vi "Listen and reply broadcast.ping.vi"(2 "error (in)":errorcluster, 3 "driplineinfolocation":string, 4 "host name":string="higgsino.physics.ucsb.edu", 5 "service name":string="monitor") -> (0 "error out":errorcluster, 1 "Log":string)   [LabVIEW 2016]
uses:
  C:/Program Files (x86)/National Instruments/LabVIEW 2016/vi.lib/Distrio/LabbitMQ/RabbitMQ.Client.dll
  Program Files (x86)/National Instruments/LabVIEW 2016/vi.lib/Distrio/LabbitMQ/RabbitMQ.Client.dll
  <vilib>/Distrio/LabbitMQ/Queue/Queue.lvclass
  <vilib>/Distrio/LabbitMQ/Connection/Connection.lvclass
panel:
  in  "stop":bool
  in  "Tab Control":enum32{"AMQP Settings", "Logger"}(tab)
  out "binding keys":string[](array[string])
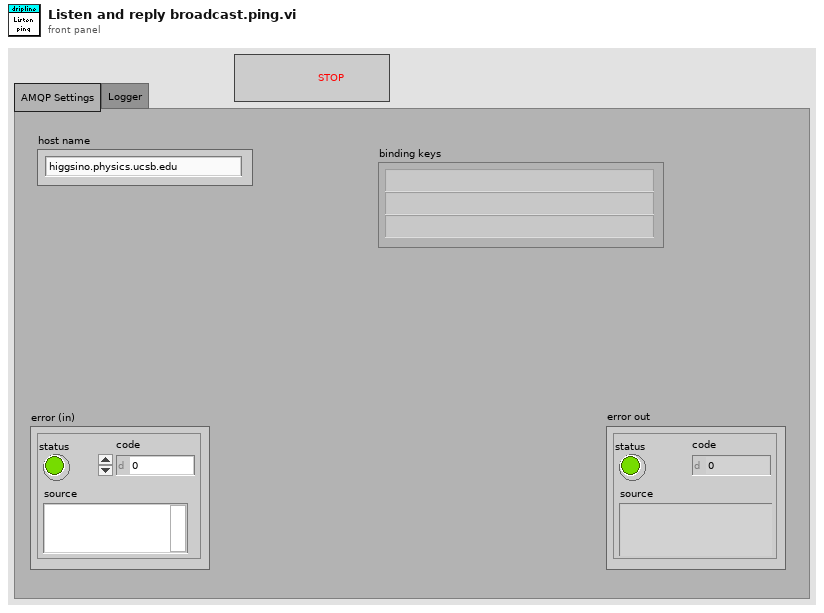
[diagram p1: front panel]
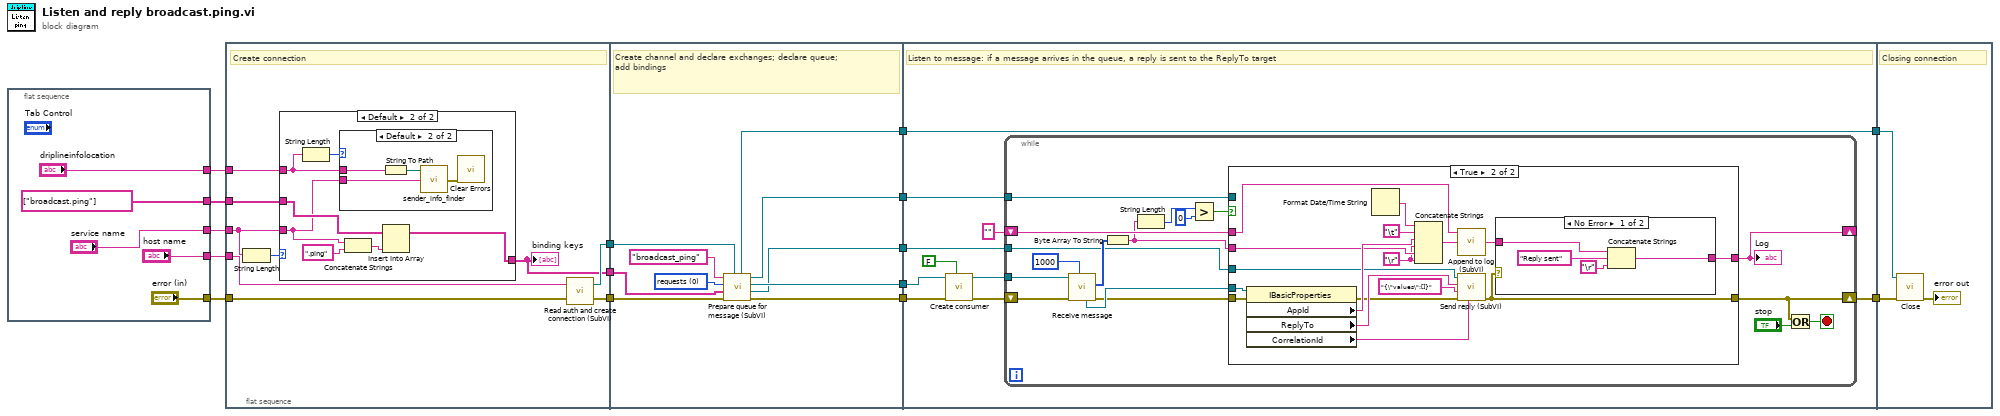
[diagram p0: block diagram]
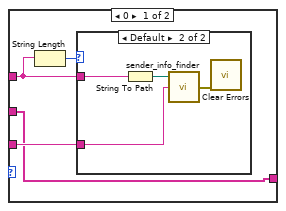
[diagram p2: hidden frame]
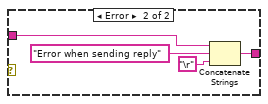
[diagram p6: hidden frame]
diagram:
  n1 = flat-sequence {
    tunnel: ["error (in)"] -> w13
    tunnel: ["host name"] -> w12
    tunnel: ["service name"] -> w4
    tunnel: ["driplineinfolocation"] -> w3
    tunnel: [string[] ["broadcast.ping"] ("broadcast.ping")] -> w1
    frame #0 {
    }
  }
  n2 = flat-sequence {
    tunnel: [w27] -> w15
    tunnel: [w26] -> w14
    tunnel: w12 -> [w29]
    tunnel: w13 -> [w28]
    tunnel: w4 -> [w24]
    tunnel: w3 -> [w25]
    tunnel: [w23] -> w2
    tunnel: w1 -> [w22]
    tunnel: w15 -> [w54]
    tunnel: w14 -> [w53]
    tunnel: [w56] -> w10
    tunnel: [w55] -> w9
    tunnel: [w52] -> w7
    tunnel: [w51] -> w6
    tunnel: [w50] -> w5
    tunnel: w2 -> [w49]
    tunnel: [w67] -> w11
    tunnel: w10 -> [w64]
    tunnel: w9 -> [w63]
    tunnel: [w62] -> w8
    tunnel: w7 -> [w62]
    tunnel: w6 -> [w61]
    tunnel: w5 -> [w60]
    tunnel: w11 -> [w114]
    tunnel: w8 -> [w113]
    frame #0 {
      # "Create connection"
      n3 = String Length(string=w24) -> (length=w21:i32)
      n4 = case shown="Default" w21 {
        tunnel: w25 -> [w30 w43]
        tunnel: w24 -> [w33 w38]
        tunnel: [w32 w40] -> w23
        tunnel: w22 -> [w32 w39]
        frame 0 {
          n5 = String Length(string=w30) -> (length=w31:i32)
          n6 = case shown="Default" w31 {
            tunnel: w33 -> [_ w37]
            tunnel: w30 -> [_ w34]
            frame 0 {
            }
            frame Default {
              n7 = String To Path(string=w34) -> (path=w36:path)
              n8 = call "sender_info_finder.vi"("service name"=w37, "file (use dialog)"=w36) -> ("error (out)"=w35:errorcluster)  [unwired: 1 in]
              n9 = call <vilib>:"Clear Errors.vi"("error in (no error)"=w35) -> ()  [unwired: 5 in, 2 out]
            }
          }
        }
        frame Default {
          n10 = String Length(string=w43) -> (length=w44:i32)
          n11 = case shown="Default" w44 {
            tunnel: w38 -> [_ w48]
            tunnel: w43 -> [_ w45]
            frame 0 {
            }
            frame Default {
              n12 = String To Path(string=w45) -> (path=w47:path)
              n13 = call "sender_info_finder.vi"("service name"=w48, "file (use dialog)"=w47) -> ("error (out)"=w46:errorcluster)  [unwired: 1 in]
              n14 = call <vilib>:"Clear Errors.vi"("error in (no error)"=w46) -> ()  [unwired: 5 in, 2 out]
            }
          }
          n15 = Concatenate Strings(w38, ".ping" ("string")) -> (w41:string)
          n16 = Insert Into Array(array=w39, new element=w41) -> (w40:string[])  [unwired: 1 in]
        }
      }
      "binding keys" <- w23
      n17 = call "Read auth and create connection (SubVI).vi"("error in (no error)"=w28, "host name"=w29) -> ("error out"=w26:errorcluster, "Connection out"=w27:refnum<class "Connection.lvclass">)
    }
    frame #1 {
      w57 = u16 0 items=["requests", "alerts"] ("exchange name")
      # "Create channel and declare exchanges; declare queue;\nadd bindings"
      n18 = call "Prepare queue for message (SubVI).vi"("Connection in"=w54, "error in (no error)"=w53, "binding key"=w49, "exchange name"=w57, "queue \nname"="broadcast_ping" ("queue name")) -> ("error out"=w55:errorcluster, "Exchange.lvclass"=w51:refnum<class "Exchange.lvclass">, "Queue out"=w56:refnum<class "Queue.lvclass">, "Channel out"=w50:refnum<class "Channel.lvclass">, "Connection out"=w52:refnum<class "Connection.lvclass">)
    }
    frame #2 {
      # "Listen to message: if a message arrives in the queue, a reply is sent to the ReplyTo target"
      n19 = call <vilib>:"Create consumer.vi"("noAck? (T)"=FALSE, "error in (no error)"=w63, "Queue in"=w64) -> ("error out"=w66:errorcluster, "Queue out"=w68:refnum<class "Queue.lvclass">)  [unwired: 7 in]
      n20 = while {
        tunnel: w68 -> [w85]
        shift-right: [w69] -> w67
        shift-left: w66 -> [w84]
        shift-right: [w81] -> _
        shift-left: "" -> [w82]
        tunnel: w61 -> [w71]
        tunnel: w60 -> [w70]
        stop <- w72 stop-if-true
        n21 = call <vilib>:"Receive message.vi"("millisecondsTimeout"=1000, "error in (no error)"=w84, "Consumer in"=w85) -> ("error out"=w79:errorcluster, "message body"=w83:u8[], "MessageProperties"=w80:refnum<k24>)  [unwired: 3 in, 3 out]
        n22 = Byte Array To String(unsigned byte array=w83) -> (string=w73:string)
        n23 = String Length(string=w73) -> (length=w76:i32)
        n24 = Greater?(x=w76, y=0) -> (0:w74:bool)
        n25 = case shown="True" w74 {
          tunnel: w82 -> [w87 w104]
          tunnel: [w87 w89] -> w81
          tunnel: w80 -> [_ w103]
          tunnel: w73 -> [_ w99]
          tunnel: w79 -> [w86 w97]
          tunnel: [w86 w91] -> w69
          tunnel: w71 -> [_ w96]
          tunnel: w70 -> [_ _]
          frame False {
          }
          frame True {
            w88 = "\r"
            n26 = property class="IBasicProperties"(reference=w103, error in=w97) -> (error out=w92:errorcluster, "AppId"=w100:string, "ReplyTo"=w95:string, "CorrelationId"=w94:string)  [unwired: 1 out]
            n27 = Format Date/Time String() -> (date/time string=w102:string)  [unwired: 3 in]
            n28 = Concatenate Strings(w102, "\t", w100, w88, w99, w88) -> (w98:string)
            n29 = call "Append to log (SubVI).vi"("to append"=w98, "log in"=w104) -> ("log out"=w90:string)  [unwired: 1 in]
            n30 = call "Send reply (SubVI).vi"("Correlation ID"=w94, "error in (no error)"=w92, "reply content"="{\"values\":[]}", "target"=w95, "Exchange.lvclass"=w96) -> ("error out"=w91:errorcluster)  [unwired: 5 in, 1 out]
            n31 = case shown="No Error" w91 {
              tunnel: w90 -> [w107 w112]
              tunnel: [w105 w109] -> w89
              frame No Error {
                n32 = Concatenate Strings(w107, "Reply sent" ("string"), "\r") -> (w105:string)
              }
              frame Error {
                n33 = Concatenate Strings(w112, "Error when sending reply" ("string"), "\r") -> (w109:string)
              }
            }
          }
        }
        "Log" <- w81
        n34 = Or(x=w69, y="stop") -> (x .or. y?=w72:bool)
      }
    }
    frame #3 {
      # "Closing connection"
      n35 = call <vilib>:"Close.vi"("error in (no error)"=w114, "Connection in"=w113) -> ("error out"=→"error out":errorcluster)  [unwired: 8 in, 1 out]
    }
  }
